vi "check&create_new_folder(SubVI).vi"(10 "업로드할 파일이름":string, 11 "version 폴더 경로":path) -> (3 "dup path":path)   [LabVIEW 2018]
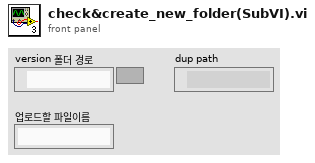
[diagram p1: front panel]
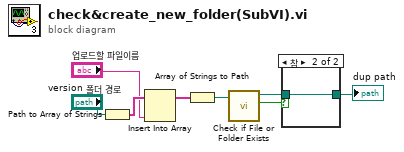
[diagram p0: block diagram]
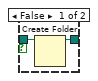
[diagram p2: hidden frame]
diagram:
  n1 = Path to Array of Strings ("경로를 문자열 배열로")(0:"version 폴더 경로") -> (2:w6:string[])  [unwired: 1 out]
  n2 = Insert Into Array(array=w6, new element="업로드할 파일이름") -> (w4:string[])  [unwired: 1 in]
  n3 = Array of Strings to Path ("문자열 배열을 경로로")(0:w4) -> (2:w5:path)  [unwired: 1 in]
  n4 = call <vilib>:"Check if File or Folder Exists.vi"("path"=w5) -> ("file or folder exists?"=w3:bool, "dup path"=w7:path)  [unwired: 8 in, 1 out]
  n5 = case shown="참" w3 {
    tunnel: w7 -> [w10 w11]
    tunnel: [w9 w11] -> w8
    frame False {
      n6 = Create Folder(path (use dialog)=w10) -> (created path=w9:path)  [unwired: 2 in, 2 out]
    }
    frame True {
    }
  }
  "dup path" <- w8
